vi "AudioTest.Play Audio.vi"() -> ()   [LabVIEW 2018]
panel:
  in  "stop":bool
  out "error out":errorcluster
  in  "device ID":u32 format="%.0x"
  in  "Audio File":path
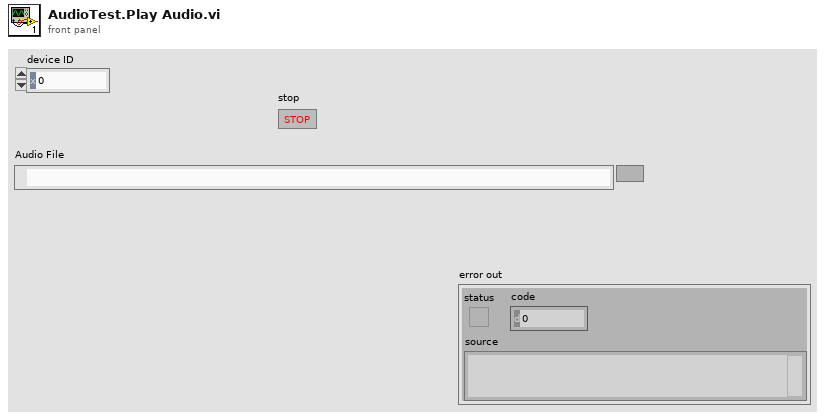
[diagram p1: front panel]
types:
  T1 = typedef "Sound Output Task ID.ctl" = u32
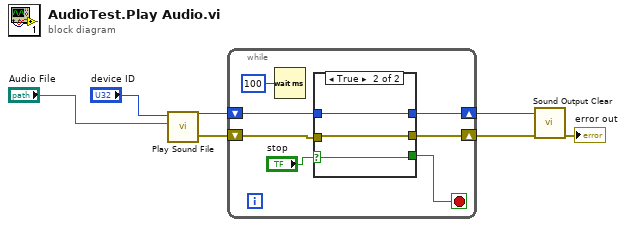
[diagram p0: block diagram]
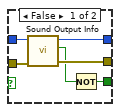
[diagram p2: hidden frame]
diagram:
  n1 = call <vilib>:"Play Sound File.vi"("path"="Audio File", "device ID"="device ID") -> ("error out"=w1:errorcluster, "task ID"=w4:T1)  [unwired: 8 in]
  n2 = while {
    shift-right: [w13] -> w3
    shift-left: w4 -> [w14]
    shift-right: [w12] -> w2
    shift-left: w1 -> [w11]
    stop <- w10 stop-if-true
    n3 = Wait (ms)(milliseconds to wait=u32 100) -> ()  [unwired: 1 out]
    n4 = case shown="True" "stop" {
      selector: "stop" -> [_ w23]
      tunnel: w14 -> [w20 w22]
      tunnel: [w19 w22] -> w13
      tunnel: [w18 w21] -> w12
      tunnel: w11 -> [w17 w21]
      tunnel: [w15 w23] -> w10
      frame False {
        n5 = call <vilib>:"Sound Output Info.vi"("error in (no error)"=w17, "task ID"=w20) -> ("error out"=w18:errorcluster, "is playing?"=w16:bool, "task ID out"=w19:T1)  [unwired: 6 in, 1 out]
        n6 = Not(x=w16) -> (.not. x?=w15:bool)
      }
      frame True {
      }
    }
  }
  n7 = call <vilib>:"Sound Output Clear.vi"("error in (no error)"=w2, "task ID"=w3) -> ("error out"=→"error out":errorcluster)  [unwired: 9 in]
